vi "WiFi HttpUpload.vi"   [LabVIEW 2014]
uses:
  QwaveSys_ESP8266/QwaveSys_ESP8266.lvlib
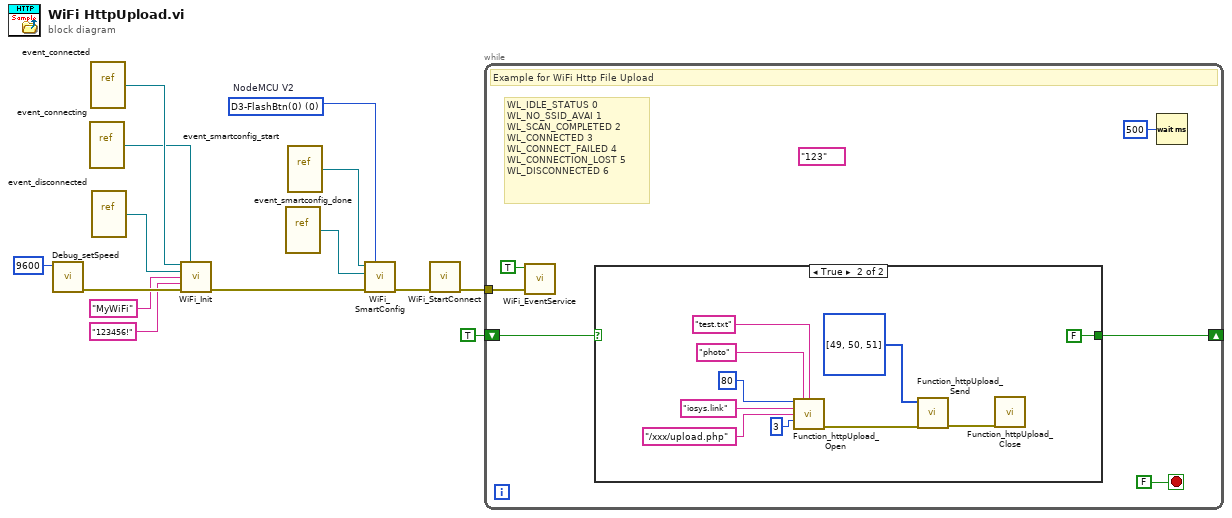
[diagram p0: block diagram]
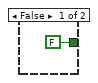
[diagram p2: hidden frame]
diagram:
  w7 = u8 0 items=["D0-(LED)-(16)"=16, "D1-SCL(5)"=5, "D2-SDA(4)"=4, "D3-FlashBtn(0)"=0, "D4-(2)"=2, "D5-SCK(14)"=14, "D6-MISO(12)"=12, "D7-MOSI(13)"=13, "D8-SS(15)"=15, "D9-TX(3)"=3, "D10-RX(1)"=1, "ADC0,(17)"=17]  # NodeMCU V2
  n1 = call "Debug_setSpeed.vi"("Speed"=u32 9600) -> ("error out"=w9:errorcluster)  [unwired: 10 in]
  n2 = vi-ref "event_connecting.vi"() -> (w4:refnum<vi>)
  n3 = vi-ref "event_connected.vi"() -> (w5:refnum<vi>)
  n4 = vi-ref "event_disconnected.vi"() -> (w3:refnum<vi>)
  n5 = call "WiFi_Init.vi"("connected"=w5, "connecting"=w4, "disconnected"=w3, "SSID"="MyWiFi", "PASSPHARSE"="123456!", "error in (no error)"=w9) -> ("error out"=w14:errorcluster)  [unwired: 9 in]
  n6 = vi-ref "event_smartconfig_done.vi"() -> (w10:refnum<vi>)
  n7 = vi-ref "event_smartconfig_start.vi"() -> (w11:refnum<vi>)
  n8 = call "WiFi_SmartConfig.vi"("Smart Config Enter Pin"=w7, "error in (no error)"=w14, "smartconfig_done"=w10, "smartconfig_start"=w11) -> ("error out"=w13:errorcluster)  [unwired: 7 in]
  n9 = call "WiFi_StartConnect.vi"("error in (no error)"=w13) -> ("error out"=w12:errorcluster)  [unwired: 10 in]
  n10 = while {
    tunnel: w12 -> [w19]
    shift-right: [w15] -> _
    shift-left: TRUE ("wait for connected (True)") -> [w16]
    stop <- FALSE stop-if-true
    (unwired) "123"
    # "WL_IDLE_STATUS\t0\nWL_NO_SSID_AVAI\t1\nWL_SCAN_COMPLETED\t2\nWL_CONNECTED\t3\nWL_CONNECT_FAILED\t4\nWL_CONNECTION_LOST\t5\nWL_DISCONNECTED\t6"
    # "Example for WiFi Http File Upload"
    n11 = call "WiFi_EventService.vi"("error in (no error)"=w19, "wait for connected (True)"=TRUE) -> ()  [unwired: 8 in, 2 out]
    n12 = case shown="True" w16 {
      tunnel: [FALSE ("wait for connected (True)") FALSE ("wait for connected (True)")] -> w15
      frame False {
      }
      frame True {
        n13 = call "Function_httpUpload_Open.vi"("Port"=i8 80, "Name"="photo", "Filename"="test.txt", "Host"="iosys.link", "URI"="/xxx/upload.php", "Upload Lenght"=u32 3) -> ("error out"=w24:errorcluster)  [unwired: 9 in]
        n14 = call "Function_httpUpload_Send.vi"("error in (no error)"=w24, "DATA"=u8[] [49, 50, 51]) -> ("error out"=w23:errorcluster)  [unwired: 9 in]
        n15 = call "Function_httpUpload_Close.vi"("error in (no error)"=w23) -> ()  [unwired: 10 in, 1 out]
      }
    }
    n16 = Wait (ms)(milliseconds to wait=u32 500) -> ()  [unwired: 1 out]
  }
